vi "Acquire and Save.vi"(8 "error in (no error)":errorcluster, 11 "DAQ Class in":refnum<class "DAQ Class.lvclass">) -> (0 "error out":errorcluster, 3 "DAQ Class out":refnum<class "DAQ Class.lvclass">)   [LabVIEW 2014, in "DAQ Class.lvclass"]
uses:
  DAQ Class.lvclass
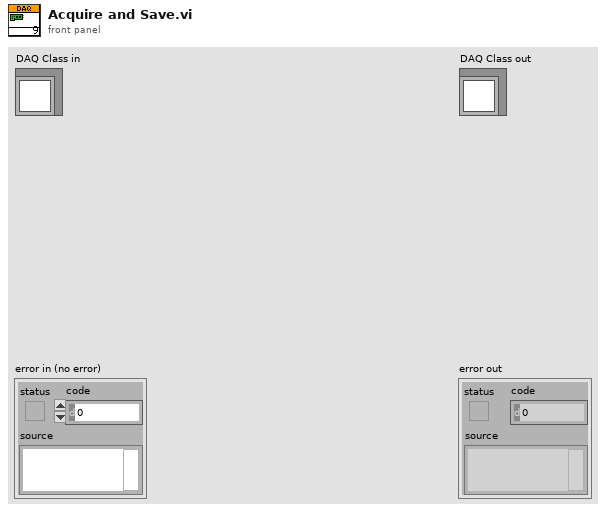
[diagram p1: front panel]
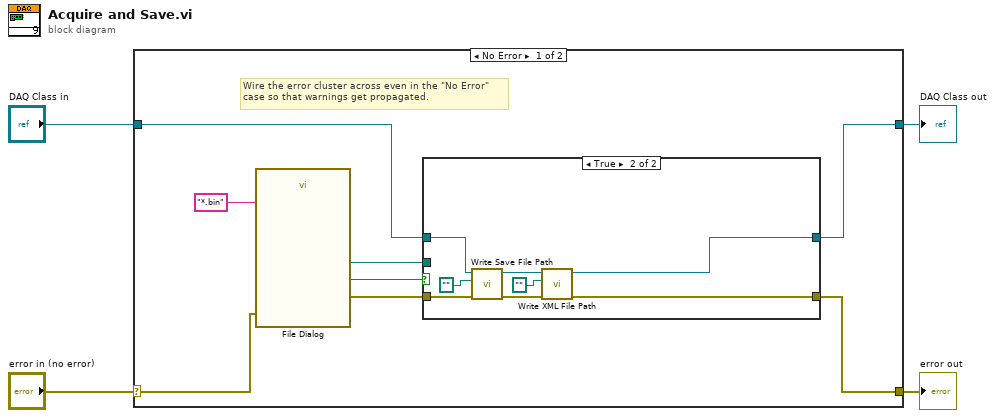
[diagram p0: block diagram]
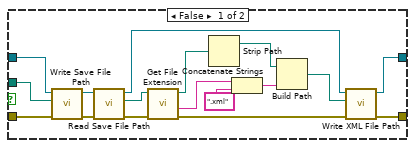
[diagram p2: hidden frame]
diagram:
  n1 = case shown="No Error" "error in (no error)" {
    selector: "error in (no error)" -> [w7 w39]
    tunnel: [w6 w39] -> w3
    tunnel: [w8 w38] -> w1
    tunnel: "DAQ Class in" -> [w9 w38]
    frame No Error {
      # "Wire the error cluster across even in the \"No Error\"\ncase so that warnings get propagated."
      n2 = call "File Dialog"("error in"=w7, "pattern (all files)"="*.bin" ("pattern label")) -> ("selected path"=w10:path, "cancelled"=w12:bool, "error out"=w11:errorcluster)  [unwired: 10 in, 1 out]
      n3 = case shown="True" w12 {
        tunnel: w11 -> [w29 w37]
        tunnel: w10 -> [w28 _]
        tunnel: w9 -> [w27 w35]
        tunnel: [w18 w30] -> w8
        tunnel: [w20 w33] -> w6
        frame False {
          n4 = call-dynamic "Write Save File Path.vi"("error in (no error)"=w29, "Save File Path"=w28, "DAQ Class in"=w27) -> ("error out"=w16:errorcluster, "DAQ Class out"=w17:refnum<class "DAQ Class.lvclass">)  [unwired: 7 in]
          n5 = call-dynamic "Read Save File Path.vi"("error in (no error)"=w16, "DAQ Class in"=w17) -> ("error out"=w15:errorcluster, "Save File Path"=w13:path, "DAQ Class out"=w14:refnum<class "DAQ Class.lvclass">)  [unwired: 7 in]
          n6 = call <vilib>:"Get File Extension.vi"("error in (no error)"=w15, "file"=w13) -> ("error out"=w21:errorcluster, "filename without extension"=w25:string, "dup file"=w26:path)  [unwired: 6 in, 1 out]
          n7 = Strip Path(path=w26) -> (stripped path=w22:path)  [unwired: 1 out]
          n8 = Concatenate Strings(w25, ".xml" ("string")) -> (w23:string)
          n9 = Build Path(base path=w22, name or relative path=w23) -> (appended path=w19:path)
          n10 = call-dynamic "Write XML File Path.vi"("error in (no error)"=w21, "XML File Path"=w19, "DAQ Class in"=w14) -> ("error out"=w20:errorcluster, "DAQ Class out"=w18:refnum<class "DAQ Class.lvclass">)  [unwired: 7 in]
        }
        frame True {
          n11 = call-dynamic "Write Save File Path.vi"("error in (no error)"=w37, "Save File Path"=path "", "DAQ Class in"=w35) -> ("error out"=w34:errorcluster, "DAQ Class out"=w31:refnum<class "DAQ Class.lvclass">)  [unwired: 7 in]
          n12 = call-dynamic "Write XML File Path.vi"("error in (no error)"=w34, "XML File Path"=path "", "DAQ Class in"=w31) -> ("error out"=w33:errorcluster, "DAQ Class out"=w30:refnum<class "DAQ Class.lvclass">)  [unwired: 7 in]
        }
      }
    }
    frame Error {
    }
  }
  "error out" <- w3
  "DAQ Class out" <- w1
